vi "Get Magnet Voltage.vi"(0 "VISA resource name":refnum<visa-resource-name>, 1 "error in":T1) -> (2 "VISA resource name out":refnum<visa-resource-name>, 3 "Instrument Responded?":bool, 4 "Magnet Voltage (V)":dbl format="%.3f", 5 "error out":T1)   [LabVIEW 2019]
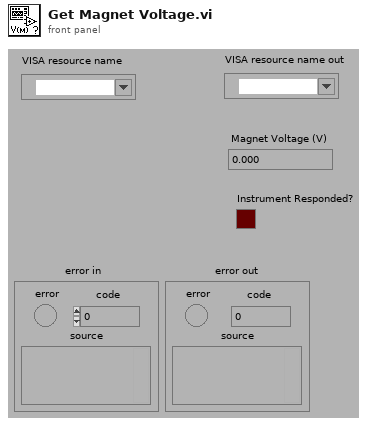
[diagram p1: front panel]
types:
  T1 = cluster{"error":bool, "code":i32, "source":string}
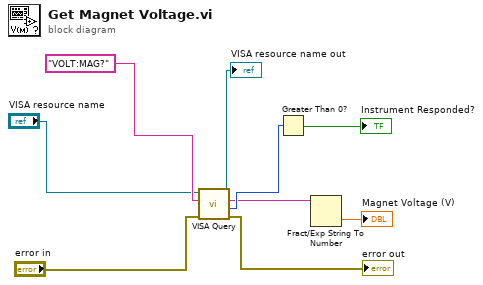
[diagram p0: block diagram]
diagram:
  n1 = call "VISA Query.vi"("error in (no error)"="error in", "Command"="VOLT:MAG?", "VISA resource name"="VISA resource name") -> ("error out"=→"error out":errorcluster, "Bytes Read"=w5:i32, "Response"=w3:string, "VISA resource name out"=→"VISA resource name out":refnum<visa-resource-name>)  [unwired: 4 in, 1 out]
  n2 = Greater Than 0?(x=w5) -> (x > 0?=→"Instrument Responded?":bool)
  n3 = Fract/Exp String To Number(string=w3) -> (number=→"Magnet Voltage (V)":dbl)  [unwired: 3 in, 1 out]
